vi "extrinsic_cluster2angleXY.vi"(11 "extrinsic cluster":cluster{"extrinsic":dbl[][], i32[]}) -> (2 "replacement":dbl[](array[numeric]), 3 "angle":dbl)   [LabVIEW 2017]
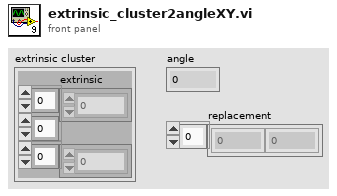
[diagram p1: front panel]
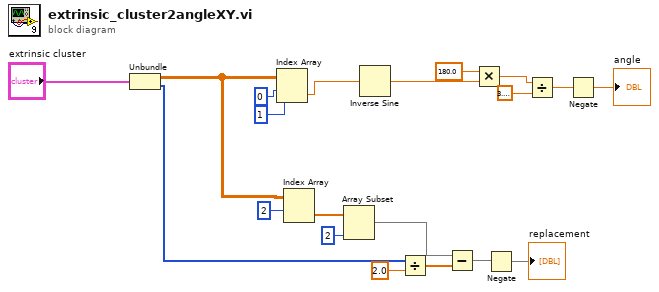
[diagram p0: block diagram]
diagram:
  n1 = Unbundle("extrinsic cluster") -> ("extrinsic"=w13:dbl[][], w18:i32[])
  n2 = Index Array(array=w13, index (row)=0, index (col)=1 ("disabled index (col)")) -> (element=w4:dbl)
  n3 = Index Array(array=w13, index (row)=2) -> (element=w12:dbl[])  [unwired: 1 in]
  n4 = Array Subset(array=w12, length=2) -> (w14:dbl[])  [unwired: 1 in]
  n5 = Inverse Sine(1:w4) -> (0:w5:dbl)
  n6 = Divide(x=w18, y=2.0) -> (x/y=w19:dbl[])
  n7 = Subtract(x=w14, y=w19) -> (x-y=w15:dbl[])
  n8 = Multiply(x=180.0, y=w5) -> (x*y=w7:dbl)
  n9 = Negate(x=w15) -> (-x=→"replacement":dbl[])
  n10 = Divide(x=w7, y=3.141592653589793) -> (x/y=w9:dbl)
  n11 = Negate(x=w9) -> (-x=→"angle":dbl)
